vi "Create Test Configuration.vi"() -> (0 "error out":errorcluster, 1 "Names":string[](array[string]), 2 "Line Array":T1[](array[typedef]), 3 "Module Configuration":refnum<class "PID Module configuration.lvclass">, 4 "Channels":refnum<class "TBM channel.lvclass">[](array[class]), 5 "instance identifier":string)   [LabVIEW 2015, in "PID Module tests.lvlib"]
doc: "This VI creates a standard test configuration for other unit tests. It currently creates and adds one line with every datatype to the module configuration."
uses:
  PID Module tests.lvlib
  module/configuration/PID Module configuration.lvclass
  module/configuration/Line.ctl
  <vilib>/NI/Tag Bus Module Framework/channel/TBM channel.lvclass
  <vilib>/NI/Tag Bus/tag/tag descriptor.lvclass/tag descriptor.ctl
  <vilib>/NI/Tag Bus/tag/default value polymorphs/write default value Double.vi
  <vilib>/NI/Configuration Framework/serializable configuration/NISE_CEF_serializable configuration.lvclass
  <vilib>/NI/Tag Bus/tag/tag descriptor.lvclass
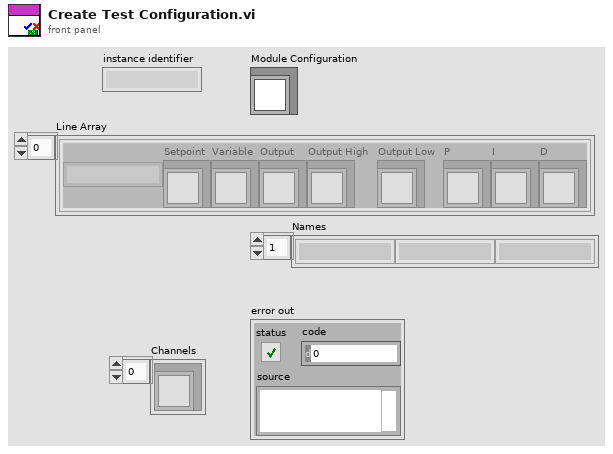
[diagram p1: front panel]
types:
  T1 = typedef "PID Module configuration.lvclass/Line.ctl" = cluster{"PID ID":string, "Setpoint":refnum<class "TBM channel.lvclass">, "Variable":refnum<class "TBM channel.lvclass">, "Output":refnum<class "TBM channel.lvclass">, "Output High":refnum<class "TBM channel.lvclass">, "Output Low":refnum<class "TBM channel.lvclass">, "P":refnum<class "TBM channel.lvclass">, "I":refnum<class "TBM channel.lvclass">, "D":refnum<class "TBM channel.lvclass">}
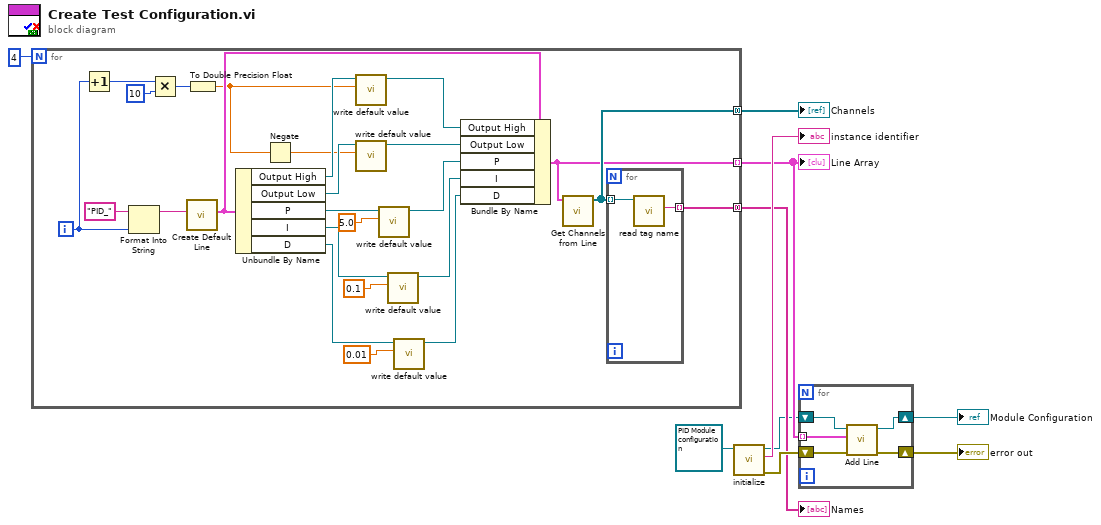
[diagram p0: block diagram]
diagram:
  n1 = for {
    N: 4 -> [_]
    tunnel: [w23] -> w6 mode=indexing
    tunnel: [w34] -> w2 mode=concatenating
    tunnel: [w33] -> w7 mode=concatenating
    i -> [w30]
    n2 = Increment(x=w30) -> (x+1=w29:i32)
    n3 = Format Into String(initial string="PID_", w30) -> (resulting string=w32:string)  [unwired: 2 in, 1 out]
    n4 = Multiply(x=w29, y=10) -> (x*y=w21:i32)
    n5 = call "Create Default Line.vi"("Line Name"=w32) -> ("Default Line"=w31:T1)  [unwired: 10 in]
    n6 = To Double Precision Float(number=w21) -> (double precision float=w20:dbl)
    n7 = Unbundle By Name(w31) -> ("Output High"=w24:refnum<class "TBM channel.lvclass">, "Output Low"=w27:refnum<class "TBM channel.lvclass">, "P"=w19:refnum<class "TBM channel.lvclass">, "I"=w16:refnum<class "TBM channel.lvclass">, "D"=w12:refnum<class "TBM channel.lvclass">)
    n8 = Negate(x=w20) -> (-x=w22:dbl)
    n9 = call-poly <vilib>:"write default value.vi"("default value"=w20, "system tag in"=w24) -> ("system tag out"=w25:refnum<class "TBM channel.lvclass">)  [unwired: 8 in, 1 out]
    n10 = call-poly <vilib>:"write default value.vi"("default value"=w22, "system tag in"=w27) -> ("system tag out"=w26:refnum<class "TBM channel.lvclass">)  [unwired: 8 in, 1 out]
    n11 = call-poly <vilib>:"write default value.vi"("default value"=5.0, "system tag in"=w19) -> ("system tag out"=w18:refnum<class "TBM channel.lvclass">)  [unwired: 8 in, 1 out]
    n12 = call-poly <vilib>:"write default value.vi"("default value"=0.1, "system tag in"=w16) -> ("system tag out"=w15:refnum<class "TBM channel.lvclass">)  [unwired: 8 in, 1 out]
    n13 = call-poly <vilib>:"write default value.vi"("default value"=0.01, "system tag in"=w12) -> ("system tag out"=w11:refnum<class "TBM channel.lvclass">)  [unwired: 8 in, 1 out]
    n14 = Bundle By Name(cluster=w31, "Output High"=w25, "Output Low"=w26, "P"=w18, "I"=w15, "D"=w11) -> (w23:T1)
    n15 = call "Get Channels from Line.vi"("Line"=w23) -> ("Channels"=w34:refnum<class "TBM channel.lvclass">[])  [unwired: 10 in]
    n16 = for {
      tunnel: w34 -> [w37] mode=indexing
      tunnel: [w36] -> w33 mode=indexing
      n17 = call <vilib>:"read tag name.vi"("system tag in"=w37) -> ("name"=w36:string)  [unwired: 8 in, 2 out]
    }
  }
  "Names" <- w7
  "Line Array" <- w6
  "Channels" <- w2
  n18 = call <vilib>:"initialize.vi"("configuration in"=refnum<class "PID Module configuration.lvclass"> refnum ("tag bus configurable plugin module configuration")) -> ("error out"=w8:errorcluster, "identifier"=→"instance identifier":string, "configuration out"=w3:refnum<class "PID Module configuration.lvclass">)  [unwired: 8 in]
  n19 = for {
    tunnel: w6 -> [w38] mode=indexing
    shift-right: [w41] -> w5
    shift-left: w3 -> [w42]
    shift-right: [w39] -> w10
    shift-left: w8 -> [w40]
    n20 = call "Add Line.vi"("error in"=w40, "Line"=w38, "PID Module 2 configuration in"=w42) -> ("error out"=w39:errorcluster, "PID Module 2 configuration out"=w41:refnum<class "PID Module configuration.lvclass">)  [unwired: 6 in, 1 out]
  }
  "error out" <- w10
  "Module Configuration" <- w5
